vi "Default Colors.vi"() -> (7 "Default Colors":u32[](array[colorbox])=[16777215, 16719378, 0, 0, 0, 0, 0, 0, 0, 0, 0, 0, 0, 0, 16448250])   [LabVIEW 2020, in "VolatusGUIElements.lvlib" / "HistorianCharting.lvclass"]
uses:
  HistorianCharting.lvclass
  HistorianCharting.lvclass/HistorianCharting.ctl
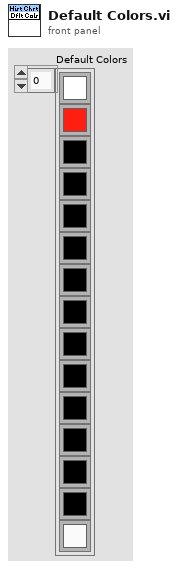
[diagram p1: front panel]
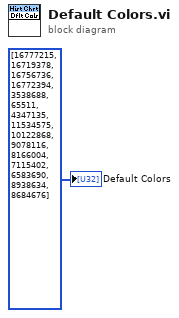
[diagram p0: block diagram]
diagram:
  "Default Colors" <- u32[] [16777215, 16719378, 16756736, 16772394, 3538688, 65511, 4347135, 11534575, 10122868, 9078116, 8166004, 7115402, 6583690, 8938634, 8684676]
